vi "robo_call.vi"(2 "错误输入（无错误）":errorcluster, 3 "mode":i32=-1, 4 "cycle":i32=1, 5 "page":i32, 6 "ax":i32, 7 "VISA资源名称":refnum<visa-resource-name>) -> (0 "错误输出":errorcluster, 1 "VISA资源名称输出":refnum<visa-resource-name>)   [LabVIEW 2017]
panel:
  # "cycle"
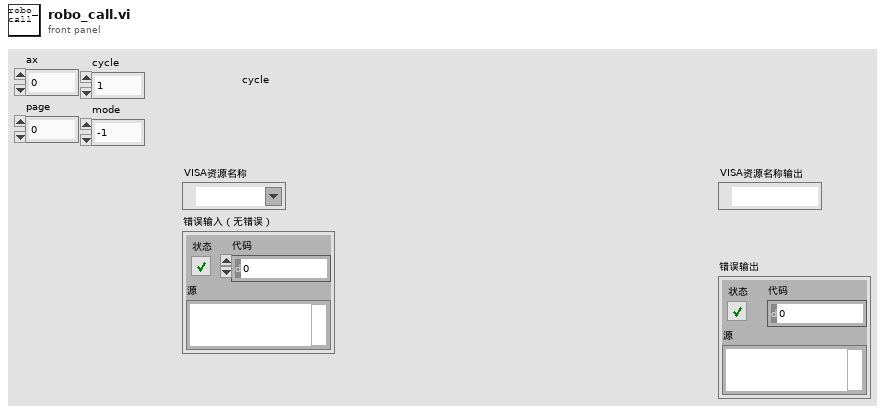
[diagram p1: front panel]
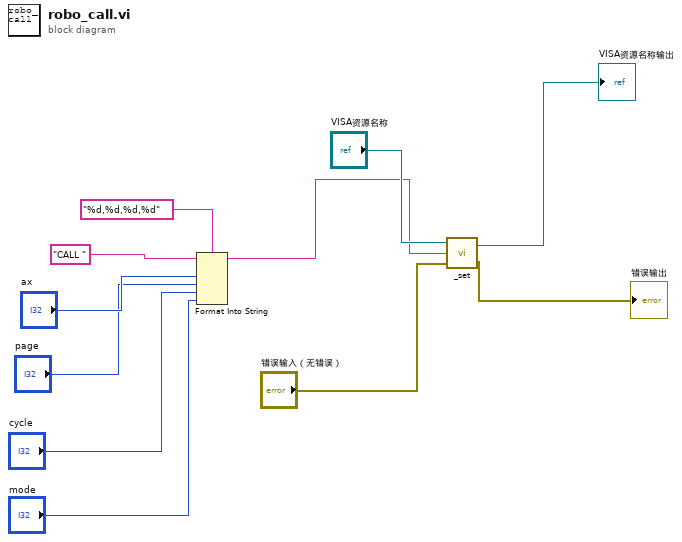
[diagram p0: block diagram]
diagram:
  n1 = Format Into String(format string="%d,%d,%d,%d" ("格式字符串"), initial string="CALL " ("初始字符串"), "ax", "page", "cycle", "mode") -> (resulting string=w6:string)  [unwired: 1 in, 1 out]
  n2 = call "_set.vi"("错误输入（无错误）"="错误输入（无错误）", "写入缓冲区"=w6, "连接ID"="VISA资源名称") -> ("错误输出"=→"错误输出":errorcluster, "连接ID输出"=→"VISA资源名称输出":refnum<k5>)
